vi "Test.vi"() -> ()   [LabVIEW 2016]
doc: "This VI is called when test mode begins, and will automatically be terminated when it ends. You can add manual or automatic tests and invoke them from the dashboard."
uses:
  <vilib>/Analysis/1siggen.llb/Ramp Pattern by Samples.vi
  SubSystems/Drive/Drive System.lvlib
  <vilib>/Analysis/NI_AALBase.lvlib
panel:
  in  "Tab Control":T1(tab)
  in  "End (V)":dbl=1.0 min=-1.0 max=1.0 step=0.02
  in  "Start (V)":dbl=-1.0 min=-1.0 max=1.0 step=0.02
  in  "Loop Rate (Hz)":i32=4 min=2 step=1
  out "Waveform Chart":T2(graph)={"[0]"=0.0, "[1]"=0.0, "[2]"=0.0, "[3]"=0.0, "[4]"=0.0, "[5]"=0.0, "[6]"=0.0, "[7]"=0.0, "[8]"=0.0, "[9]"=0.0, "[10]"=0.0, "[11]"=0.0, "[12]"=0.0, "[13]"=0.0, "[14]"=0.0, "[15]"=0.0, "[16]"=12.35}
  in  "stop":bool
  out "Waveform Chart 2":dbl[](graph)
  in  "Flappy":i32(slide) scale=0.0..270.0
  in  "Camera":i32(slide) scale=0.0..270.0
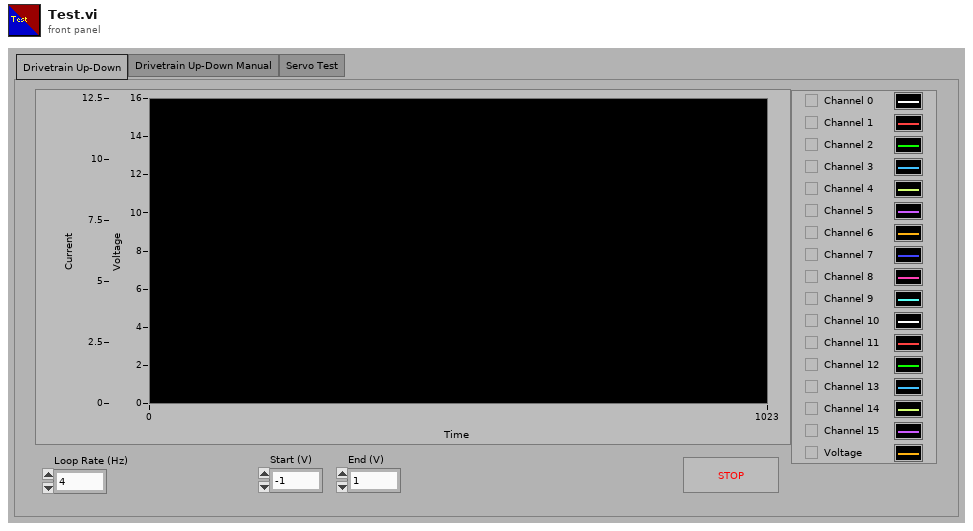
[diagram p1: front panel]
types:
  T1 = enum32{"Drivetrain Up-Down", "Drivetrain Up-Down Manual", "Servo Test"}
  T2 = cluster{"[0]":dbl, "[1]":dbl, "[2]":dbl, "[3]":dbl, "[4]":dbl, "[5]":dbl, "[6]":dbl, "[7]":dbl, "[8]":dbl, "[9]":dbl, "[10]":dbl, "[11]":dbl, "[12]":dbl, "[13]":dbl, "[14]":dbl, "[15]":dbl, "[16]":dbl}
  T3 = typedef "WPI_ServoDeviceRef.ctl" = cluster{"DeviceStatus":errorcluster, "PWM Channel":T4, "DeadBand":T5}
  T4 = typedef "FPGA_DIOPWMChannel.ctl" = enum8{"PWM 0", "PWM 1", "PWM 2", "PWM 3", "PWM 4", "PWM 5", "PWM 6", "PWM 7", "PWM 8", "PWM 9", "PWM MXP 0", "PWM MXP 1", "PWM MXP 2", "PWM MXP 3", "PWM MXP 4", "PWM MXP 5", "PWM MXP 6", "PWM MXP 7", "PWM MXP 8", "PWM MXP 9", "Invalid"}
  T5 = typedef "WPI_PWMDeadband.ctl" = cluster{"Name":string, "maxPositivePwm":i32, "minPositivePwm":i32, "centerPwm":i32, "maxNegativePwm":i32, "minNegativePwm":i32, "angularRange":u16}
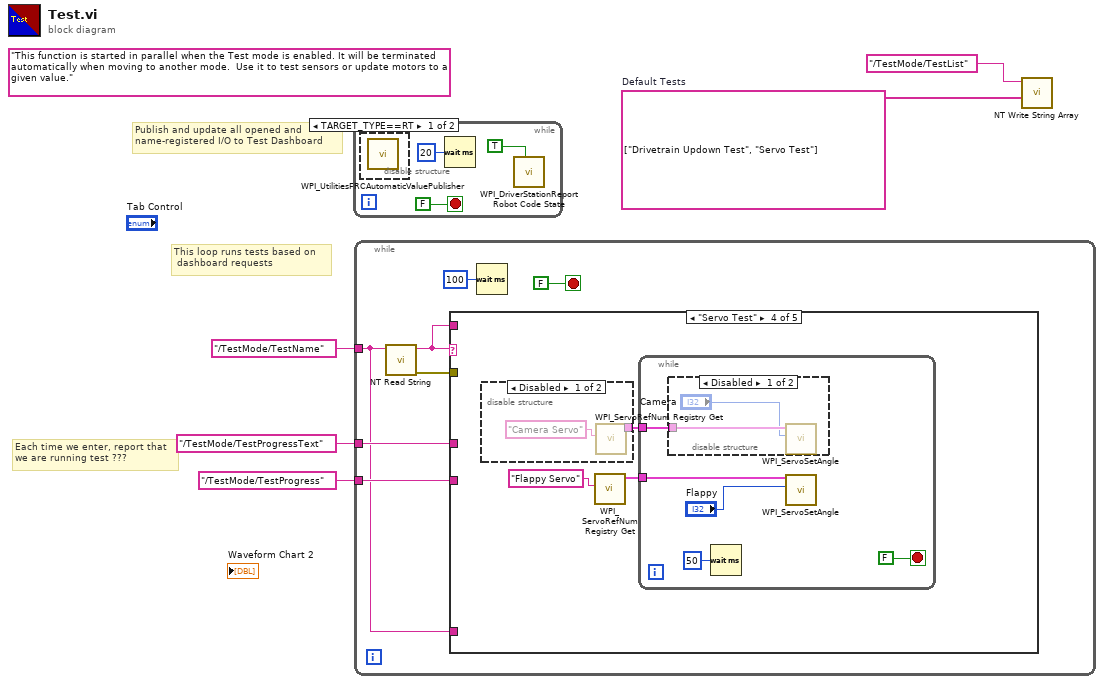
[diagram p0: block diagram]
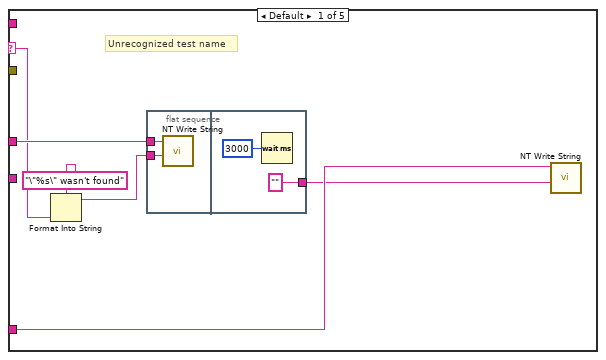
[diagram p3: hidden frame]
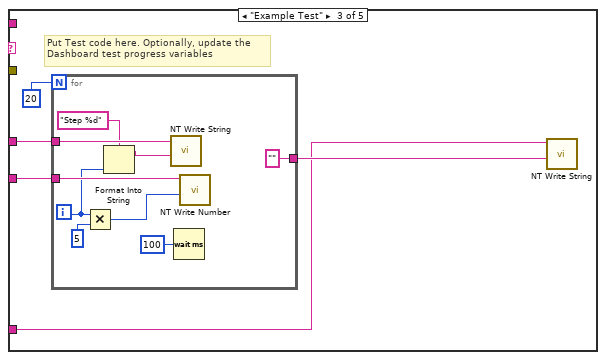
[diagram p5: hidden frame]
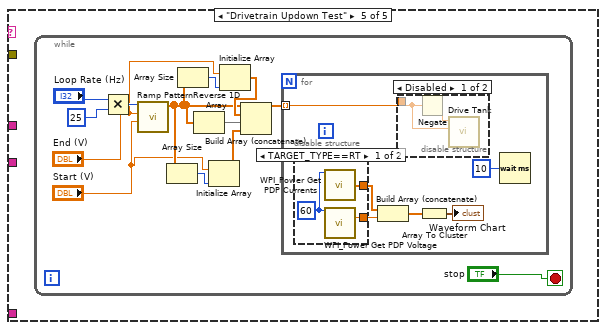
[diagram p8: hidden frame]
diagram:
  w2 = string[] ["Drivetrain Updown Test", "Servo Test"]  # Default Tests
  (unwired) "This function is started in parallel when the Test mode is enabled. It will be terminated automatically when moving to another mode.  Use it to test sensors or update motors to a given value."
  # "This loop runs tests based on \n dashboard requests"
  # "Publish and update all opened and\nname-registered I/O to Test Dashboard"
  # "Each time we enter, report that\nwe are running test ???"
  n1 = while {
    stop <- FALSE stop-if-true
    n2 = disable-structure shown="TARGET_TYPE==RT" {
      frame condition #0 (active) {
        n3 = call <vilib>:"WPI_UtilitiesFRCAutomaticValuePublisher.vi"() -> ()  [unwired: 12 in]
      }
      frame condition #1 {
      }
    }
    n4 = Wait (ms)(milliseconds to wait=u32 20) -> ()  [unwired: 1 out]
    n5 = call <vilib>:"WPI_DriverStationReport Robot Code State.vi"("Test"=TRUE ("Autonomous")) -> ()  [unwired: 10 in, 1 out]
  }
  n6 = while {
    tunnel: "/TestMode/TestName" ("Name") -> [w10]
    tunnel: "/TestMode/TestProgressText" ("Name") -> [w13]
    tunnel: "/TestMode/TestProgress" ("Name") -> [w12]
    stop <- FALSE stop-if-true
    n7 = call <vilib>:"NT Read String.vi"("Name"=w10) -> ("error out"=w9:errorcluster, "String"=w11:string)  [unwired: 9 in]
    n8 = case shown="\"Servo Test\"" w11 {
      selector: w11 -> [w20 _ _ _ _]
      tunnel: w10 -> [w17 _ w26 _ _]
      tunnel: w13 -> [w21 _ w29 _ _]
      tunnel: w12 -> [_ _ w30 _ _]
      tunnel: w11 -> [_ _ _ _ _]
      tunnel: w9 -> [_ _ _ _ _]
      frame Default {
        # "Unrecognized test name"
        n9 = Format Into String(format string="\"%s\" wasn't found" ("Name"), w20) -> (resulting string=w19:string)  [unwired: 2 in, 1 out]
        n10 = flat-sequence {
          tunnel: w21 -> [w22]
          tunnel: w19 -> [w23]
          tunnel: ["" ("Name")] -> w16
          frame #0 {
            n11 = call <vilib>:"NT Write String.vi"("String"=w23, "Name"=w22) -> ()  [unwired: 9 in, 1 out]
          }
          frame #1 {
            n12 = Wait (ms)(milliseconds to wait=u32 3000) -> ()  [unwired: 1 out]
          }
        }
        n13 = call <vilib>:"NT Write String.vi"("String"=w16, "Name"=w17) -> ()  [unwired: 9 in, 1 out]
      }
      frame "" {
        # "No test to run"
      }
      frame "Example Test" {
        # "Put Test code here. Optionally, update the\nDashboard test progress variables"
        n14 = for {
          N: 20 -> [_]
          tunnel: w30 -> [w39]
          tunnel: w29 -> [w37]
          tunnel: ["" ("String")] -> w27
          i -> [w34]
          n15 = Multiply(x=w34, y=u32 5 ("milliseconds to wait")) -> (x*y=w35:u32)
          n16 = Format Into String(format string="Step %d", w34) -> (resulting string=w32:string)  [unwired: 2 in, 1 out]
          n17 = call <vilib>:"NT Write String.vi"("String"=w32, "Name"=w37) -> ()  [unwired: 9 in, 1 out]
          n18 = Wait (ms)(milliseconds to wait=u32 100) -> ()  [unwired: 1 out]
          n19 = call <vilib>:"NT Write Number.vi"("Numeric"=w35, "Name"=w39) -> ()  [unwired: 9 in, 1 out]
        }
        n20 = call <vilib>:"NT Write String.vi"("String"=w27, "Name"=w26) -> ()  [unwired: 9 in, 1 out]
      }
      frame "Servo Test" {
        n21 = disable-structure shown="Disabled" {
          disable-tunnel: [w44 _] -> w42
          frame Disabled {
            n22 = call <vilib>:"WPI_ServoRefNum Registry Get.vi"("refnum name"="Camera Servo") -> ("ServoDeviceRef"=w44:T3)  [unwired: 9 in, 1 out]
          }
          frame Enabled {
          }
        }
        n23 = call <vilib>:"WPI_ServoRefNum Registry Get.vi"("refnum name"="Flappy Servo") -> ("ServoDeviceRef"=w41:T3)  [unwired: 9 in, 1 out]
        n24 = while {
          tunnel: w42 -> [w46]
          tunnel: w41 -> [w47]
          stop <- FALSE stop-if-true
          n25 = disable-structure shown="Disabled" {
            disable-tunnel: w46 -> [w51 _]
            frame Disabled {
              n26 = call <vilib>:"WPI_ServoSetAngle.vi"("Angle"="Camera", "ServoDeviceRef"=w51) -> ()  [unwired: 8 in, 2 out]
            }
            frame Enabled {
            }
          }
          n27 = Wait (ms)(milliseconds to wait=u32 50) -> ()  [unwired: 1 out]
          n28 = call <vilib>:"WPI_ServoSetAngle.vi"("Angle"="Flappy", "ServoDeviceRef"=w47) -> ()  [unwired: 8 in, 2 out]
        }
      }
      frame "Drivetrain Updown Test" {
        n29 = while {
          stop <- "stop" stop-if-true
          n30 = Multiply(x="Loop Rate (Hz)", y=25) -> (x*y=w63:i32)
          n31 = call-poly <vilib>:"Ramp Pattern.vi"("start"="Start (V)", "end"="End (V)", "samples"=w63) -> ("Ramp Pattern"=w54:dbl[])  [unwired: 7 in, 1 out]
          n32 = Array Size(array=w54) -> (size(s)=w55:i32)
          n33 = Array Size(array=w54) -> (size(s)=w58:i32)
          n34 = Reverse 1D Array(array=w54) -> (reversed array=w59:dbl[])
          n35 = Initialize Array("Start (V)", w55) -> (w52:dbl[])
          n36 = Initialize Array("End (V)", w58) -> (w56:dbl[])
          n37 = Build Array (concatenate)(w54, w56, w59, w52) -> (w61:dbl[])
          n38 = for {
            tunnel: w61 -> [w66] mode=indexing
            n39 = disable-structure shown="TARGET_TYPE==RT" {
              disable-tunnel: [w75 _] -> w70
              disable-tunnel: [w74 _] -> w69
              frame condition #0 (active) {
                w73 = u8 60 ("Power Distribution Panel (0)")
                n40 = call <vilib>:"WPI_Power Get PDP Currents.vi"("Power Distribution Panel (0)"=w73) -> ("all currents (A)"=w75:dbl[])  [unwired: 12 in, 2 out]
                n41 = call <vilib>:"WPI_Power Get PDP Voltage.vi"("Power Distribution Panel (0)"=w73) -> ("voltage (V)"=w74:dbl)  [unwired: 13 in, 1 out]
              }
              frame condition #1 {
              }
            }
            n42 = Build Array (concatenate)(w70, w69) -> (w68:dbl[])
            n43 = disable-structure shown="Disabled" {
              disable-tunnel: w66 -> [w72 _]
              frame Disabled {
                n44 = Negate(x=w72) -> (-x=w71:dbl)
                n45 = call "Drive Tank.vi"("Right"=w72, "Left"=w71) -> ()  [unwired: 9 in, 1 out]
              }
              frame Enabled {
              }
            }
            n46 = Array To Cluster(array=w68) -> (cluster=→"Waveform Chart":T2)
            n47 = Wait (ms)(milliseconds to wait=u32 10) -> ()  [unwired: 1 out]
          }
        }
      }
    }
    n48 = Wait (ms)(milliseconds to wait=u32 100) -> ()  [unwired: 1 out]
  }
  n49 = call <vilib>:"NT Write String Array.vi"("String Array"=w2, "Name"="/TestMode/TestList") -> ()  [unwired: 9 in, 1 out]
